vi "Do.vi"(8 "error in (no error)":errorcluster, 10 "Actor in":refnum<class "Actor.lvclass">, 11 "Configure Alarms Msg":refnum<class "Configure Alarms Msg.lvclass">) -> (0 "error out":errorcluster, 2 "Actor out":refnum<class "Actor.lvclass">)   [LabVIEW 2016, in "LS218.lvlib" / "Configure Alarms Msg.lvclass"]
doc: "This VI delivers the message to the actor by calling the appropriate method(s) on the actor."
uses:
  Configure Alarms Msg.lvclass
  <vilib>/ActorFramework/Actor/Actor.lvclass
  C:/User/Brand/LVP/STF/Packages/CSPP_Core/Actors/CS++PVMonitor Messages/CS++PVUpdate Msg/CS++PVUpdate Msg.lvclass
  LS218/LS218.lvclass
  C:/Program Files (x86)/National Instruments/LabVIEW 2016/vi.lib/ActorFramework/Actor/Actor.lvclass
  CSPP_Core/Actors/CS++PVMonitor Messages/CS++PVUpdate Msg/CS++PVUpdate Msg.lvclass/CS++PVUpdate Msg.ctl
  CSPP_Core/Classes/CS++ProcessVariables/ProcessVariable/PV.lvclass/PV.ctl
  Configure Alarms Msg.lvclass/Configure Alarms Msg.ctl
  CSPP_Core/Classes/CS++ProcessVariables/ProcessVariable/PV.lvclass
  CSPP_Core/Actors/CS++PVMonitor Messages/CS++PVUpdate Msg/CS++PVUpdate Msg.lvclass
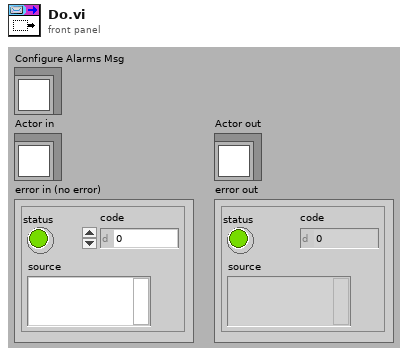
[diagram p1: front panel]
types:
  T1 = cluster{"Input (0)":i32, "Alarm Limits":cluster{"High Value (0.0000)":dbl[unit], "Low Value (0.0000)":dbl[unit], "Deadband (0.0000)":dbl[unit]}, "Boolean Alarm Controls":cluster{"Alarm (F: Alarm Disabled)":bool, "Beeper (F: Beeper Disabled)":bool, "Latching (F: Alarm Latch OFF)":bool}}
  T2 = cluster{"High Value (0.0000)":dbl[unit], "Low Value (0.0000)":dbl[unit], "Deadband (0.0000)":dbl[unit]}
  T3 = cluster{"Alarm (F: Alarm Disabled)":bool, "Beeper (F: Beeper Disabled)":bool, "Latching (F: Alarm Latch OFF)":bool}
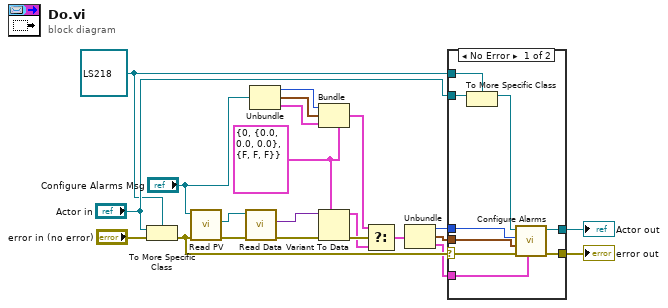
[diagram p0: block diagram]
diagram:
  w14 = T1 {"Input (0)"=0, "Alarm Limits"={"High Value (0.0000)"=0.0, "Low Value (0.0000)"=0.0, "Deadband (0.0000)"=0.0}, "Boolean Alarm Controls"={"Alarm (F: Alarm Disabled)"=FALSE, "Beeper (F: Beeper Disabled)"=FALSE, "Latching (F: Alarm Latch OFF)"=FALSE}} ("Type")
  w18 = refnum<class "LS218.lvclass"> refnum ("Actor in")
  n1 = To More Specific Class(target class=w18, reference="Actor in", error in="error in (no error)") -> (error out=w7:errorcluster)  [unwired: 1 out]
  n2 = call "Read PV.vi"("error in (no error)"=w7, "CS++PVUpdate Msg in"="Configure Alarms Msg") -> ("error out"=w17:errorcluster, "PV"=w13:refnum<class "PV.lvclass">)  [unwired: 7 in, 1 out]
  n3 = call "Read Data.vi"("error in (no error)"=w17, "PV in"=w13) -> ("error out"=w11:errorcluster, "Data"=w12:variant)  [unwired: 7 in, 1 out]
  n4 = Unbundle ("Pre-Unbundler")("Configure Alarms Msg") -> (w3:i32, w2:T2, w1:T3)
  n5 = Bundle ("Pre-Bundler")(cluster=w14, "Input (0)"=w3, "Alarm Limits"=w2, "Boolean Alarm Controls"=w1) -> (w15:T1)
  n6 = Variant To Data(error in=w11, type=w14, Variant=w12) -> (data=w9:T1, error out=w16:errorcluster)
  n7 = Select ("MainSelect")(t=w15, s=w16, f=w9) -> (s? t:f=w10:T1)
  n8 = Unbundle ("Main-Unbundler")(w10) -> ("Input (0)"=w6:i32, "Alarm Limits"=w5:T2, "Boolean Alarm Controls"=w4:T3)
  n9 = case shown="No Error" w7 {
    selector: w7 -> [w29 w33]
    tunnel: [w31 w33] -> w21
    tunnel: [w30 w32] -> w20
    tunnel: "Actor in" -> [w28 w32]
    tunnel: w18 -> [w27 _]
    tunnel: w6 -> [w25 _]
    tunnel: w5 -> [w24 _]
    tunnel: w4 -> [w23 _]
    frame No Error {
      n10 = To More Specific Class(target class=w27, reference=w28) -> (specific class reference=w26:refnum<class "LS218.lvclass">)  [unwired: 1 in, 1 out]
      n11 = call "Configure Alarms.vi"("Boolean Alarm Controls"=w23, "error in (no error)"=w29, "Alarm Limits"=w24, "Input (0)"=w25, "LS218 in"=w26) -> ("error out"=w31:errorcluster, "LS218 out"=w30:refnum<class "LS218.lvclass">)  [unwired: 5 in]
    }
    frame Error {
    }
  }
  "error out" <- w21
  "Actor out" <- w20
